vi "Host_FastOsziTest.vi"() -> ()   [LabVIEW 2012]
uses:
  <vilib>/FPGAPlugInAG/PXIe-7962R/niLvFpga_Open_PXIe-7962R.vi
  <vilib>/rvi/interface/common/dynamic/niFpgaDynamicAddResources.vi
  <vilib>/Utility/error.llb/Error Cluster From Error Code.vi
  <vilib>/rvi/errors/niLvFpgaAdjustHostInterfaceError.vi
  <vilib>/FPGAPlugInAG/Dynamic/niLvFpga_Close_Dynamic.vi
  <vilib>/rvi/interface/nirviOpenFPGA/nirviOpenFPGA.xnode
  FPGA Bitfiles/AnalogIntegratorFastOszi_NI5771_PXIe-7962R.lvbitx
  <vilib>/rvi/interface/nirviReadWriteControl/nirviReadWriteControl.xnode
  <vilib>/rvi/interface/nirviMethod/nirviMethod.xnode
  <vilib>/rvi/interface/nirviCloseFPGA/nirviCloseFPGA.xnode
  <vilib>/rvi/interface/Simulation/niFpgaSimulationCallBeginRW.vi
  NiFpgaLv.dll
  <vilib>/FPGAPlugInAG/Dynamic/niLvFpga_ReadFifo_Dynamic.vi
  <vilib>/rvi/errors/niLvFpgaMergeErrorWithErrorCode.vi
  <vilib>/Analysis/NI_AALPro.lvlib
panel:
  in  "Repetition Rate":bool=TRUE
  in  "Baseline Subtract":u8=16
  out "NOT Crosstalk":dbl format="%0.2f"
  out "Crosstalk":dbl format="%0.2f"
  in  "Save?":bool
  out "time to draw(ms) 2":i32=1000
  out "Area 1":picture
  in  "sized scatter plot cosmetics 2":T1={"min size"=1, "max size"=5, "maps to max size"=5, "color array"=[16711680, 65280, 255, 16776960, 16737792, 65535]}
  in  "cartesian axis attributes 2":T2={"x minimum"=1.0, "x maximum"=500.0, "x log?"=FALSE, "x precision"=1, "x format"=enum."Decimal", "y minimum"=60.0, "y maximum"=740.0, "y log?"=FALSE, "y precision"=1, "y format"=enum."Decimal"} {"x minimum" format="%0.2f"; "x maximum" format="%0.2f"; "y minimum" format="%0.2f"; "y maximum" format="%0.2f"}
  in  "?":u16(ring)=4 items=["Points", "Squares", "Circles", "Sized Squares", "Sized-Colored Squares", "Min-Max Lines"]
  in  "line color 2":u32(colorbox)=39168
  in  "text color 2":u32(colorbox)=65280
  in  "plot color 2":u32(colorbox)=16776960
  out "time to draw(ms)":i32=1000
  out "Area 2":picture
  in  "sized scatter plot cosmetics":T1={"min size"=1, "max size"=5, "maps to max size"=5, "color array"=[16711680, 65280, 255, 16776960, 16737792, 65535]}
  in  "cartesian axis attributes":T2={"x minimum"=1.0, "x maximum"=500.0, "x log?"=FALSE, "x precision"=1, "x format"=enum."Decimal", "y minimum"=60.0, "y maximum"=740.0, "y log?"=FALSE, "y precision"=1, "y format"=enum."Decimal"} {"x minimum" format="%0.2f"; "x maximum" format="%0.2f"; "y minimum" format="%0.2f"; "y maximum" format="%0.2f"}
  in  "?":u16(ring)=4 items=["Points", "Squares", "Circles", "Sized Squares", "Sized-Colored Squares", "Min-Max Lines"]
  in  "line color":u32(colorbox)=39168
  in  "text color":u32(colorbox)=65280
  in  "plot color":u32(colorbox)=16776960
  out "PMT histogram":T3(graph)
  out "Mean NOT pulse length":dbl format="%0.2f"
  out "Mean pulse length":dbl format="%0.2f"
  out "NOT Laser pulse length histogram":T3(graph)
  out "Laser pulse length histogram":T3(graph)
  out "Laser (Trigger In)":i16[](graph)
  in  "Samples per Pixels":u32=10000
  out "IO Module\\AI Over Range":bool
  out "PMT (AI 0)":u8[](graph)
  # "Sampling at 1.5GHz => 0.66 ns sampling interval"
  # "40MHz"
  # "80MHz"
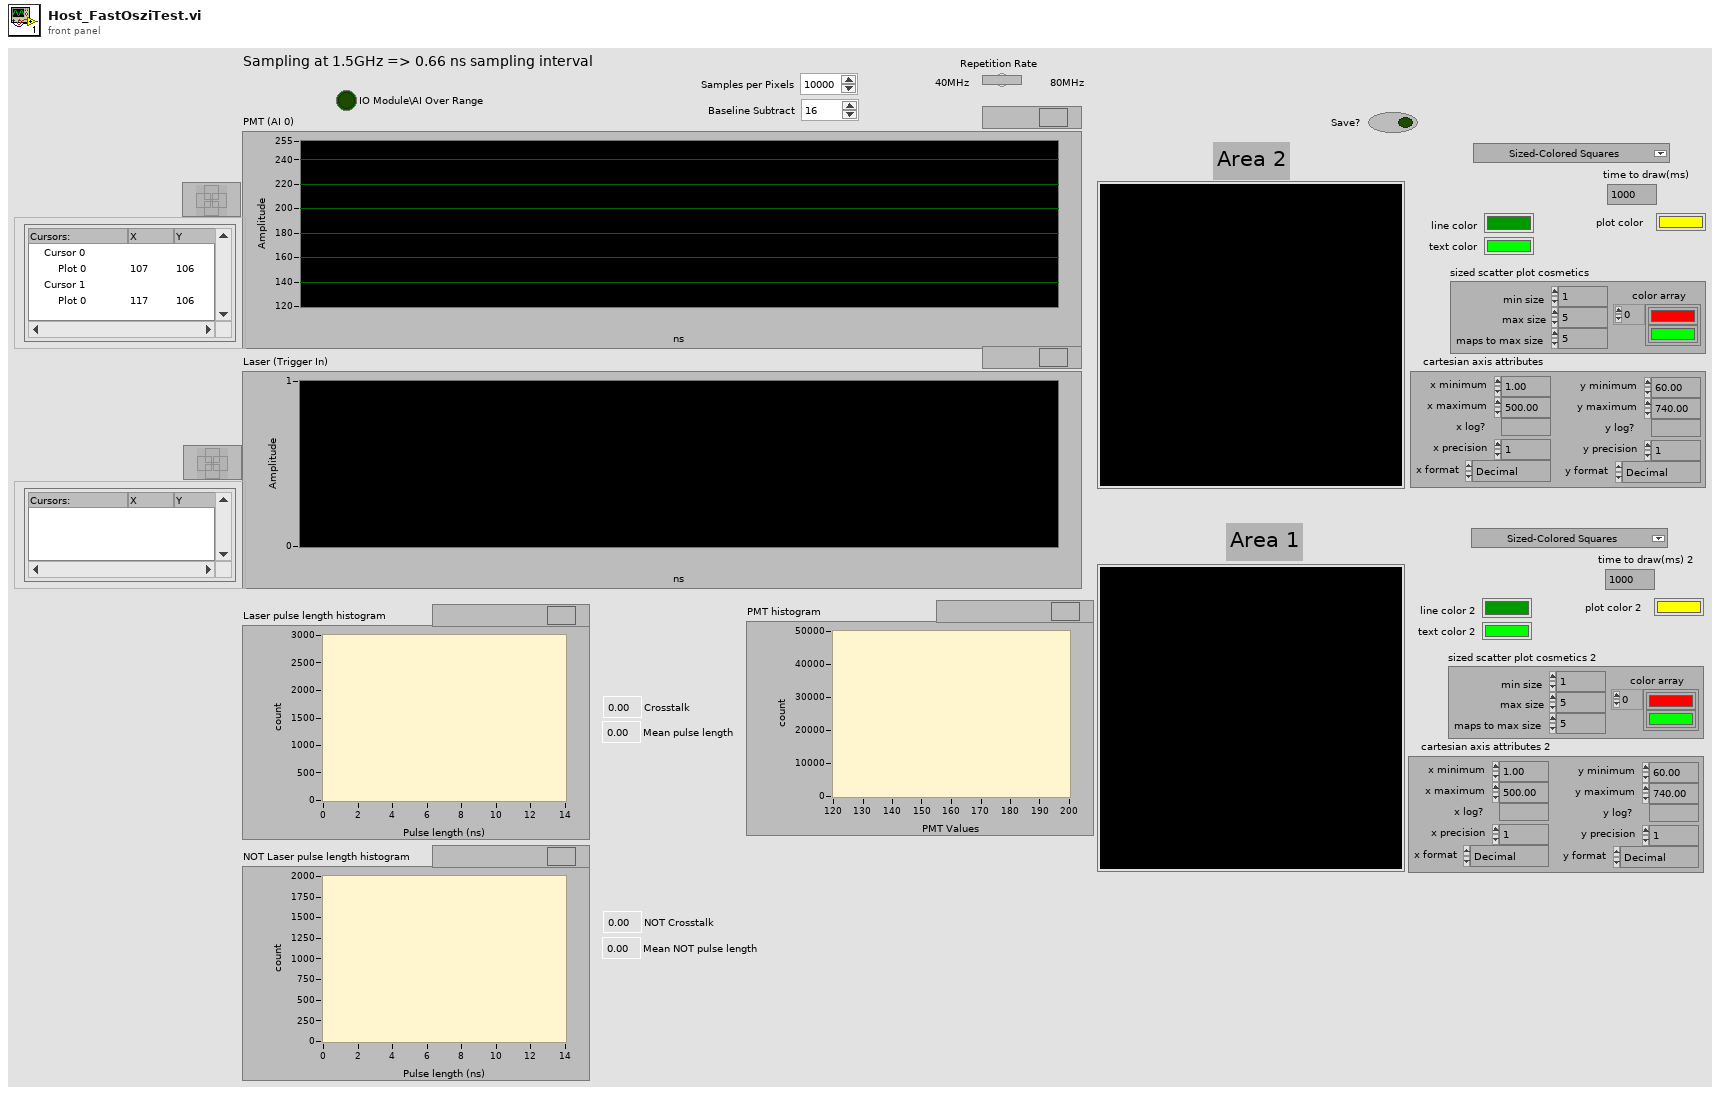
[diagram p1: front panel]
types:
  T1 = cluster{"min size":i16, "max size":i16, "maps to max size":i16, "color array":u32[]}
  T2 = cluster{"x minimum":dbl, "x maximum":dbl, "x log?":bool, "x precision":u8, "x format":enum8{"Decimal", "Scientific", "Engineering", "Binary", "Octal", "Hex"}, "y minimum":dbl, "y maximum":dbl, "y log?":bool, "y precision":u8, "y format":enum8{"Decimal", "Scientific", "Engineering", "Binary", "Octal", "Hex"}}
  T3 = cluster{"X Values":dbl[], "Histogram: h(x)":i32[]}
  T4 = typedef "LVBoundsTypeDef.ctl" = cluster{"Width":u32, "Height":u32}
  T5 = cluster{"line color 2":u32, "text color 2":u32, "tick length":i16, "not crossing axes":bool, "no grids":bool}
  T6 = cluster{"plot color 2":u32, i32, "baseline(not used for these plots)":i16}
  T7 = cluster{cluster{i32, i32, "Width":u32, "Height":u32}, "cartesian axis attributes 2":cluster{"x minimum":dbl, "x maximum":dbl, "x log?":bool, "x precision":u8, "x format":enum8{"Decimal", "Scientific", "Engineering", "Binary", "Octal", "Hex"}, "y minimum":dbl, "y maximum":dbl, "y log?":bool, "y precision":u8, "y format":enum8{"Decimal", "Scientific", "Engineering", "Binary", "Octal", "Hex"}}, cluster{"line color 2":u32, "text color 2":u32, "tick length":i16, "not crossing axes":bool, "no grids":bool}, cluster{"plot color 2":u32, i32, "baseline(not used for these plots)":i16}, "sized scatter plot cosmetics 2":cluster{"min size":i16, "max size":i16, "maps to max size":i16, "color array":u32[]}}
  T8 = cluster{"line color":u32, "text color":u32, "tick length":i16, "not crossing axes":bool, "no grids":bool}
  T9 = cluster{"plot color":u32, i32, "baseline(not used for these plots)":i16}
  T10 = cluster{cluster{i32, i32, "Width":u32, "Height":u32}, "cartesian axis attributes":cluster{"x minimum":dbl, "x maximum":dbl, "x log?":bool, "x precision":u8, "x format":enum8{"Decimal", "Scientific", "Engineering", "Binary", "Octal", "Hex"}, "y minimum":dbl, "y maximum":dbl, "y log?":bool, "y precision":u8, "y format":enum8{"Decimal", "Scientific", "Engineering", "Binary", "Octal", "Hex"}}, cluster{"line color":u32, "text color":u32, "tick length":i16, "not crossing axes":bool, "no grids":bool}, cluster{"plot color":u32, i32, "baseline(not used for these plots)":i16}, "sized scatter plot cosmetics":cluster{"min size":i16, "max size":i16, "maps to max size":i16, "color array":u32[]}}
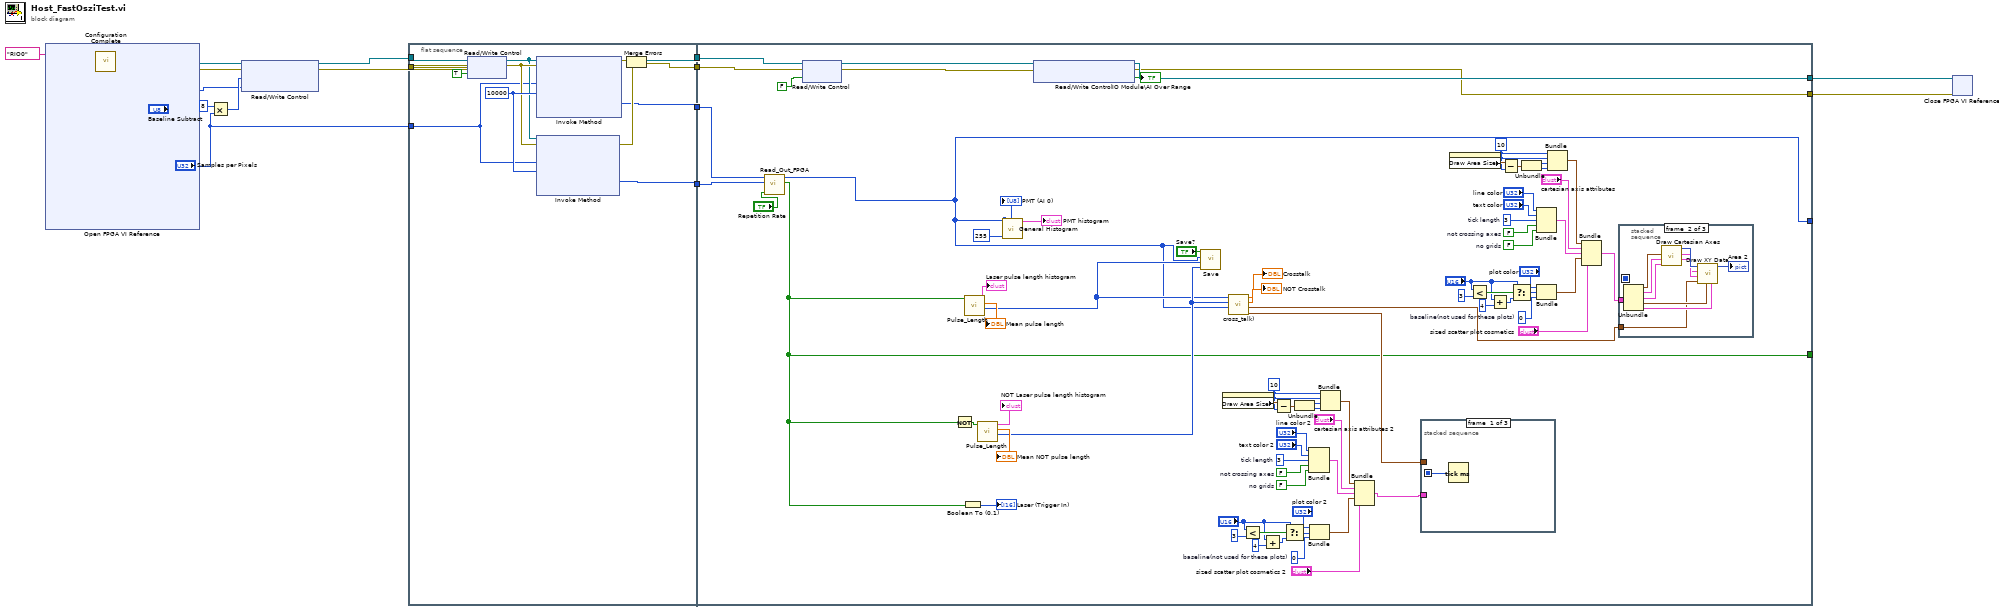
[diagram p0: block diagram]
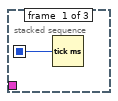
[diagram p2: hidden frame]
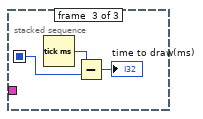
[diagram p3: hidden frame]
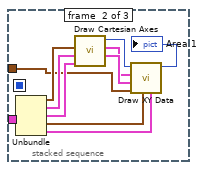
[diagram p4: hidden frame]
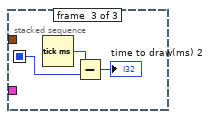
[diagram p5: hidden frame]
diagram:
  n1 = xnode "Open FPGA VI Reference"("resource name"=tag "RIO0") -> ("FPGA VI Reference Out"=w11:refnum<k20>, "error out"=w16:errorcluster)  [unwired: 1 in]
  n2 = call "Configuration Complete.vi"("error in"=w16, "FPGA VI Reference In"=w11) -> ("error out"=w14:errorcluster, "FPGA VI Reference Out"=w15:refnum<k20>)  [unwired: 7 in, 1 out]
  n3 = Multiply(x=u32 8, y="Samples per Pixels") -> (x*y=w7:u32)
  n4 = xnode "Read/Write Control"("FPGA VI Reference In"=w15, "error in"=w14, "Samples to acquire"=w7, "Baseline U8"="Baseline Subtract") -> ("FPGA VI Reference Out"=w12:refnum<k20>, "error out"=w13:errorcluster)
  n5 = flat-sequence {
    tunnel: w13 -> [w22]
    tunnel: w12 -> [w24]
    tunnel: [w23] -> w4
    tunnel: [w19] -> w3
    tunnel: [w21] -> w2
    tunnel: [w18] -> w1
    tunnel: "Samples per Pixels" -> [w20]
    tunnel: [w106] -> w10
    tunnel: [w105] -> w9
    tunnel: [w33] -> _
    tunnel: [w32] -> _
    tunnel: w4 -> [w100]
    tunnel: w3 -> [w103]
    tunnel: w2 -> [w101]
    tunnel: w1 -> [w102]
    frame #0 {
      w30 = 10000 ("Timeout (ms)")
      n6 = xnode "Read/Write Control"("FPGA VI Reference In"=w24, "error in"=w22, "Acquire"=TRUE) -> ("FPGA VI Reference Out"=w26:refnum<k20>, "error out"=w27:errorcluster)
      n7 = xnode "Invoke Method"("FPGA VI Reference In"=w26, "error in"=w27, "Number of Elements"=w20, "Timeout (ms)"=w30) -> ("FPGA VI Reference Out"=w23:refnum<k20>, "error out"=w28:errorcluster, "Data"=w19:u64[])  [unwired: 1 out]
      n8 = xnode "Invoke Method"("FPGA VI Reference In"=w26, "error in"=w27, "Number of Elements"=w20, "Timeout (ms)"=w30) -> ("error out"=w29:errorcluster, "Data"=w18:u8[])  [unwired: 2 out]
      n9 = Merge Errors(w28, w29) -> (w21:errorcluster)
    }
    frame #1 {
      w43 = i16 0  # baseline(not used for these plots)
      w50 = FALSE  # not crossing axes
      w51 = i16 3  # tick length
      w49 = FALSE  # no grids
      w54 = 10
      w66 = i16 0  # baseline(not used for these plots)
      w73 = FALSE  # not crossing axes
      w74 = i16 3  # tick length
      w72 = FALSE  # no grids
      w77 = 10
      n10 = call "Read_Out_FPGA.vi"("Repetition Rate"="Repetition Rate", "U8ReadFIFO"=w102, "U64ReadFIFO"=w103) -> ("Trigger"=w32:bool[], "PMT Signal"=w33:u8[])  [unwired: 7 in]
      "PMT (AI 0)" <- w33
      n11 = xnode "Read/Write Control"("FPGA VI Reference In"=w100, "error in"=w101, "Acquire"=FALSE) -> ("FPGA VI Reference Out"=w98:refnum<k20>, "error out"=w99:errorcluster)
      n12 = Not(x=w32) -> (.not. x?=w95:bool[])
      n13 = Boolean To (0,1)(Boolean=w32) -> (0, 1=→"Laser (Trigger In)":i16[])
      n14 = call "Pulse_Length.vi"("Trigger"=w32) -> ("Rising Index"=w84:i32[], "Mean Pulse Length"=→"Mean pulse length":dbl, "Histogram Graph"=→"Laser pulse length histogram":T3)  [unwired: 8 in]
      n15 = call "Pulse_Length.vi"("Trigger"=w95) -> ("Rising Index"=w87:i32[], "Mean Pulse Length"=→"Mean NOT pulse length":dbl, "Histogram Graph"=→"NOT Laser pulse length histogram":T3)  [unwired: 8 in]
      n16 = call <vilib>:"General Histogram.vi"("X"=w33, "# bins"=255) -> ("Histogram Graph"=→"PMT histogram":T3)  [unwired: 9 in, 4 out]
      n17 = xnode "Read/Write Control"("FPGA VI Reference In"=w98, "error in"=w99) -> ("FPGA VI Reference Out"=w106:refnum<k20>, "error out"=w105:errorcluster, "IO Module\\AI Over Range"=→"IO Module\\AI Over Range":bool)
      n18 = call "Save.vi"("Rising Index 1"=w87, "Rising Index 2"=w84, "PMT (AI 0)"=w33, "Save?"="Save?") -> ()  [unwired: 8 in]
      n19 = property on="Area 1" class="Pict"() -> ("Draw Area Size"=w81:T4)  [unwired: 2 in, 2 out]
      n20 = call "cross_talk).vi"("Array"=w33, "Rising Index 2"=w87, "Rising Index"=w84) -> ("data 2"=w83:cluster{"x":dbl, "y":dbl}[], "data"=w82:cluster{"x":dbl, "y":dbl}[], "x/y 2"=→"NOT Crosstalk":dbl, "x/y"=→"Crosstalk":dbl)  [unwired: 5 in]
      n21 = Less?(x="?", y=3) -> (x < y?=w71:bool)
      n22 = Add(x="?", y=4) -> (x+y=w69:i32)
      n23 = Subtract(x=w81, y=w77) -> (x-y=w80:T4)
      n24 = Select(t="?", s=w71, f=w69) -> (s? t:f=w67:i32)
      n25 = Unbundle(w80) -> ("Width"=w78:u32, "Height"=w79:u32)
      n26 = Bundle("line color 2"="line color 2", "text color 2"="text color 2", "tick length"=w74, "not crossing axes"=w73, "no grids"=w72) -> (w61:T5)  [unwired: 1 in]
      n27 = Bundle("plot color 2"="plot color 2", w67, "baseline(not used for these plots)"=w66) -> (w62:T6)  [unwired: 1 in]
      n28 = Bundle(w77, w77, "Width"=w78, "Height"=w79) -> (w59:cluster{i32, i32, "Width":u32, "Height":u32})  [unwired: 1 in]
      n29 = Bundle(w59, "cartesian axis attributes 2"="cartesian axis attributes 2", w61, w62, "sized scatter plot cosmetics 2"="sized scatter plot cosmetics 2") -> (w35:T7)  [unwired: 1 in]
      n30 = stacked-sequence {
        seq-local: [w122 _ _] -> [_ _ w135]
        tunnel: w35 -> [_ w127 _]
        tunnel: w83 -> [_ w123 _]
        frame #0 {
          n31 = Tick Count (ms)() -> (millisecond timer value=w122:u32)
        }
        frame #1 {
          n32 = Unbundle(w127) -> (w128:cluster{i32, i32, "Width":u32, "Height":u32}, "cartesian axis attributes 2"=w129:T2, w130:T5, w125:T6, "sized scatter plot cosmetics 2"=w124:T1)
          n33 = call <vilib>:"Draw Cartesian Axes.vi"("grid cosmetics"=w130, "axis attributes"=w129, "bounding rect"=w128) -> ("y scale factors"=w132:cluster{"a":dbl, "b":dbl, "log?":bool}, "x scale factors"=w131:cluster{"a":dbl, "b":dbl, "log?":bool}, "new picture"=w133:picture)  [unwired: 6 in]
          n34 = call <vilib>:"Draw XY Data.vi"("[sized scatter plot cosmetics]"=w124, "xy cosmetics"=w125, "xy data"=w123, "y scale factors"=w132, "x scale factors"=w131, "picture"=w133) -> ("new picture"=→"Area 1":picture)  [unwired: 5 in]
        }
        frame #2 {
          n35 = Tick Count (ms)() -> (millisecond timer value=w136:u32)
          n36 = Subtract(x=w136, y=w135) -> (x-y=→"time to draw(ms) 2":u32)
        }
      }
      n37 = property on="Area 2" class="Pict"() -> ("Draw Area Size"=w58:T4)  [unwired: 2 in, 2 out]
      n38 = Less?(x="?", y=3) -> (x < y?=w48:bool)
      n39 = Add(x="?", y=4) -> (x+y=w46:i32)
      n40 = Subtract(x=w58, y=w54) -> (x-y=w57:T4)
      n41 = Select(t="?", s=w48, f=w46) -> (s? t:f=w44:i32)
      n42 = Unbundle(w57) -> ("Width"=w55:u32, "Height"=w56:u32)
      n43 = Bundle("line color"="line color", "text color"="text color", "tick length"=w51, "not crossing axes"=w50, "no grids"=w49) -> (w38:T8)  [unwired: 1 in]
      n44 = Bundle("plot color"="plot color", w44, "baseline(not used for these plots)"=w43) -> (w39:T9)  [unwired: 1 in]
      n45 = Bundle(w54, w54, "Width"=w55, "Height"=w56) -> (w36:cluster{i32, i32, "Width":u32, "Height":u32})  [unwired: 1 in]
      n46 = Bundle(w36, "cartesian axis attributes"="cartesian axis attributes", w38, w39, "sized scatter plot cosmetics"="sized scatter plot cosmetics") -> (w34:T10)  [unwired: 1 in]
      n47 = stacked-sequence {
        seq-local: [w107 _ _] -> [_ _ w120]
        tunnel: w34 -> [_ w112 _]
        tunnel: w82 -> [_ w108 _]
        frame #0 {
          n48 = Tick Count (ms)() -> (millisecond timer value=w107:u32)
        }
        frame #1 {
          n49 = Unbundle(w112) -> (w113:cluster{i32, i32, "Width":u32, "Height":u32}, "cartesian axis attributes"=w114:T2, w115:T8, w110:T9, "sized scatter plot cosmetics"=w109:T1)
          n50 = call <vilib>:"Draw Cartesian Axes.vi"("grid cosmetics"=w115, "axis attributes"=w114, "bounding rect"=w113) -> ("y scale factors"=w117:cluster{"a":dbl, "b":dbl, "log?":bool}, "x scale factors"=w116:cluster{"a":dbl, "b":dbl, "log?":bool}, "new picture"=w118:picture)  [unwired: 6 in]
          n51 = call <vilib>:"Draw XY Data.vi"("[sized scatter plot cosmetics]"=w109, "xy cosmetics"=w110, "xy data"=w108, "y scale factors"=w117, "x scale factors"=w116, "picture"=w118) -> ("new picture"=→"Area 2":picture)  [unwired: 5 in]
        }
        frame #2 {
          n52 = Tick Count (ms)() -> (millisecond timer value=w121:u32)
          n53 = Subtract(x=w121, y=w120) -> (x-y=→"time to draw(ms)":u32)
        }
      }
    }
  }
  n54 = xnode "Close FPGA VI Reference"("FPGA VI Reference In"=w10, "error in"=w9) -> ()  [unwired: 1 out]
